vi "Update ref dwell.vi"(8 "error in (no error)":errorcluster, 11 "Ref_dwellTime":sgl) -> (0 "error out":errorcluster)   [LabVIEW 2020]
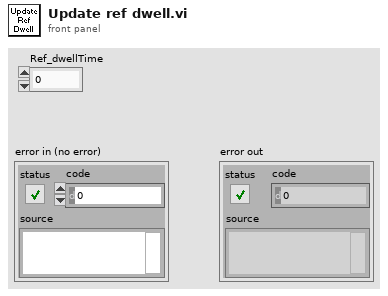
[diagram p1: front panel]
types:
  T1 = typedef "Reference_Globals.ctl" = cluster{"Refrence data path":path, "Reference Rectangle":i16[][], "AOL Z":dbl, "No of pixels in a miniscan ":i32[], "Threshold":i16[], "No of miniscans":i32[], "Full Frame Size":u16, "Reference Image":T2, "dwelltime":dbl, "Zoom":dbl, "Field of View":dbl, "Z Step":i8, "Z pixels":i32, "Z Lines":u8, "Z Ignore":u8, "Laser":u8}
  T2 = typedef "IMAQ Image.ctl" = refnum<image>
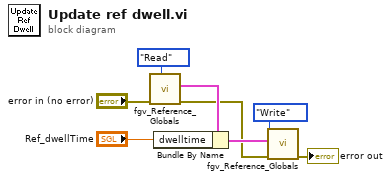
[diagram p0: block diagram]
diagram:
  n1 = call "fgv_Reference_Globals.vi"("error in (no error)"="error in (no error)", "Function"=enum16{"Intialize", "Write", "Read", "Clear"}."Read") -> ("error out"=w3:errorcluster, "Reference Data"=w6:T1)  [unwired: 8 in]
  n2 = Bundle By Name(cluster=w6, "dwelltime"="Ref_dwellTime") -> (w7:T1)
  n3 = call "fgv_Reference_Globals.vi"("error in (no error)"=w3, "Reference Data"=w7, "Function"=enum16{"Intialize", "Write", "Read", "Clear"}."Write") -> ("error out"=→"error out":errorcluster)  [unwired: 7 in, 1 out]
